vi "File.Move File to New Folder.vi"(7 "Action":enum16{"Move", "Copy"}(ring), 8 "error in":errorcluster, 10 "Destination Folder":path, 11 "Source File Path":path) -> (0 "error out":errorcluster, 3 "New Path":path)   [LabVIEW 2024]
uses:
  Errors/Error.Error Code List.ctl
  Errors.lvlib
  File Utils.lvlib
panel:
  out "Dir":bool
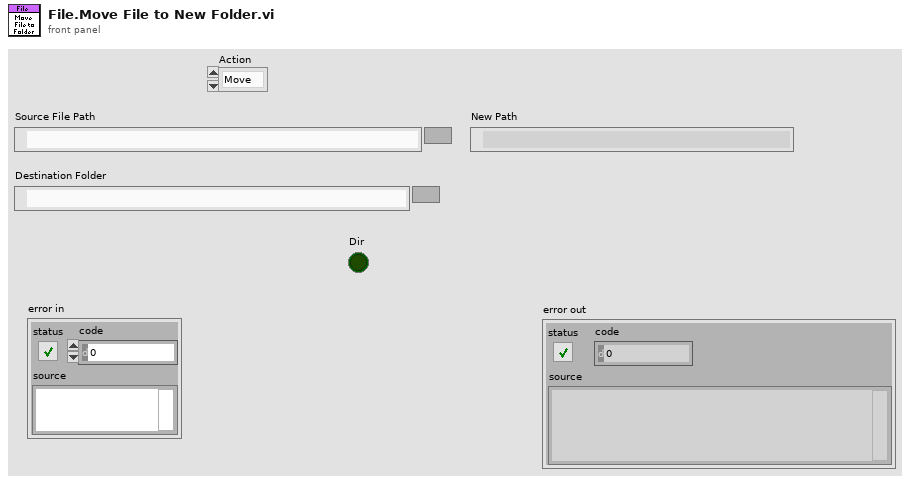
[diagram p1: front panel]
types:
  T1 = typedef "EQMF.lvlib/Errors.lvlib/Error.Error Code List.ctl" = i32
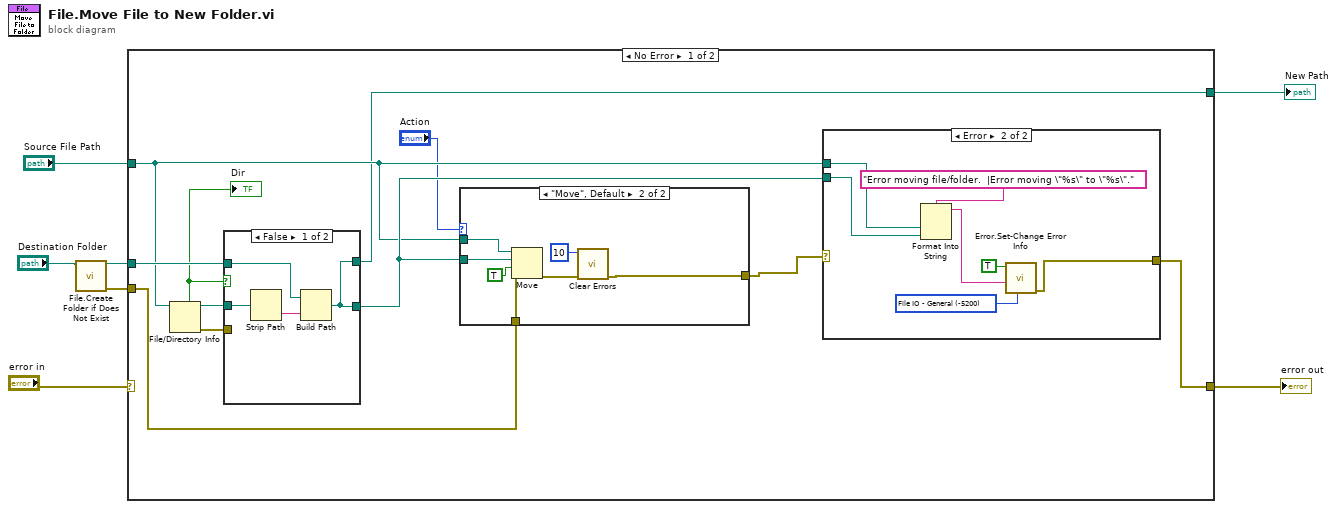
[diagram p0: block diagram]
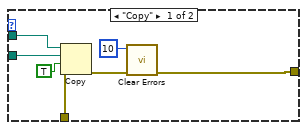
[diagram p2: hidden frame]
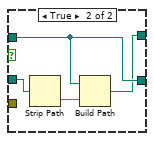
[diagram p3: hidden frame]
diagram:
  n1 = call "File.Create Folder if Does Not Exist.vi"("Path"="Destination Folder") -> ("error out"=w1:errorcluster, "Dup Path"=w3:path)  [unwired: 8 in, 1 out]
  n2 = case shown="No Error" "error in" {
    selector: "error in" -> [_ w48]
    tunnel: w3 -> [w18 _]
    tunnel: "Source File Path" -> [w15 _]
    tunnel: [w16 w48] -> w6
    tunnel: [w9 _] -> w5
    tunnel: w1 -> [w10 _]
    frame No Error {
      n3 = File/Directory Info(path=w15) -> (path out=w13:path, directory=w12:bool, error out=w11:errorcluster)  [unwired: 1 in, 4 out]
      "Dir" <- w12
      n4 = case shown="False" w12 {
        tunnel: w18 -> [w35 w38]
        tunnel: [w33 w38] -> w17
        tunnel: w13 -> [w34 w39]
        tunnel: w11 -> [_ _]
        tunnel: [w33 w37] -> w9
        frame False {
          n5 = Strip Path(path=w34) -> (name=w36:string)  [unwired: 1 out]
          n6 = Build Path(base path=w35, name or relative path=w36) -> (appended path=w33:path)
        }
        frame True {
          n7 = Strip Path(path=w39) -> (name=w40:string)  [unwired: 1 out]
          n8 = Build Path(base path=w38, name or relative path=w40) -> (appended path=w37:path)
        }
      }
      n9 = case shown="\"Move\", Default" "Action" {
        tunnel: w17 -> [w25 w32]
        tunnel: w15 -> [w24 w31]
        tunnel: [w19 w26] -> w14
        tunnel: w10 -> [w23 w30]
        frame "Copy" {
          n10 = Copy(8:w23, 9:TRUE ("overwrite (F)"), 10:w25, 11:w24) -> (0:w22:errorcluster)  [unwired: 1 in, 2 out]
          n11 = call <vilib>:"Clear Errors.vi"("error in (no error)"=w22, "specific error code to clear (0: all)"=10) -> ("error out"=w19:errorcluster)  [unwired: 4 in, 1 out]
        }
        frame "Move", Default {
          n12 = Move(source path=w31, error in=w30, 9:TRUE ("overwrite (F)"), 10:w32) -> (error out=w29:errorcluster)  [unwired: 1 in, 2 out]
          n13 = call <vilib>:"Clear Errors.vi"("error in (no error)"=w29, "specific error code to clear (0: all)"=10) -> ("error out"=w26:errorcluster)  [unwired: 4 in, 1 out]
        }
      }
      n14 = case shown="Error" w14 {
        tunnel: w15 -> [_ w47]
        tunnel: w17 -> [_ w46]
        tunnel: [_ w41] -> w16
        frame No Error {
        }
        frame Error {
          w43 = T1 -5200 items=["No Error"=0, "Abort"=-2, "Misc"=-5000, "Fixture Error"=-5100, "File IO - General"=-5200, "FIle IO - Config Error"=-5201, "Instrument - General"=-5300, "Instrument - Serial Com"=-5301, "Instrument - Camera"=-5302, "Instrument - PS"=-5303, "Instrument - Oscilloscope"=-5304, "Instrument - Function Gen"=-5305, "Instrument - Load"=-5306, "Instrument - Meter"=-5307, "Instrument - Power Control"=-5308, "Instrument - Motion"=-5309, "Instrument - RF"=-5310, "System Exe"=-5400, "Image Processing"=-5500, "Communication"=-5600, "Script - Syntax Error"=-6000, "Script - Invalid Name or Param"=-6100, "Script - Timeout"=-6200, "Invalid Data"=-6300, "FW Update Error"=-6500] ("Std Code")
          n15 = Format Into String(format string="Error moving file/folder.  |Error moving \"%s\" to \"%s\".", w47, w46) -> (resulting string=w42:string)  [unwired: 2 in, 1 out]
          n16 = call "Error.Set-Change Error Info.vi"("Std Code"=w43, "Description"=w42, "Set Error"=TRUE) -> ("error out"=w41:errorcluster)  [unwired: 8 in]
        }
      }
    }
    frame Error {
    }
  }
  "New Path" <- w5
  "error out" <- w6
